vi "Powerstage_Relay_test_v1.vi"() -> ()   [LabVIEW 2022 SP3]
uses:
  <vilib>/DAQmx/read.llb/DAQmx Read (Digital 1D Bool NChan 1Samp 1Line).vi
  <vilib>/DAQmx/miscellaneous.llb/DAQmx Fill In Error Info.vi
panel:
  out "error out":errorcluster
  in  "error in (no error)":errorcluster
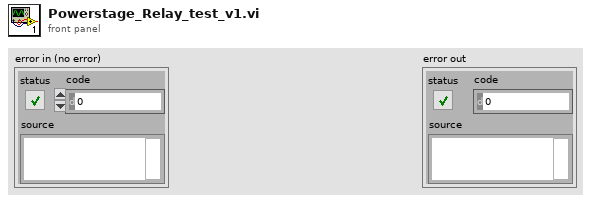
[diagram p1: front panel]
types:
  T1 = cluster{"Set":string, "State on":string, "State off":string}[]
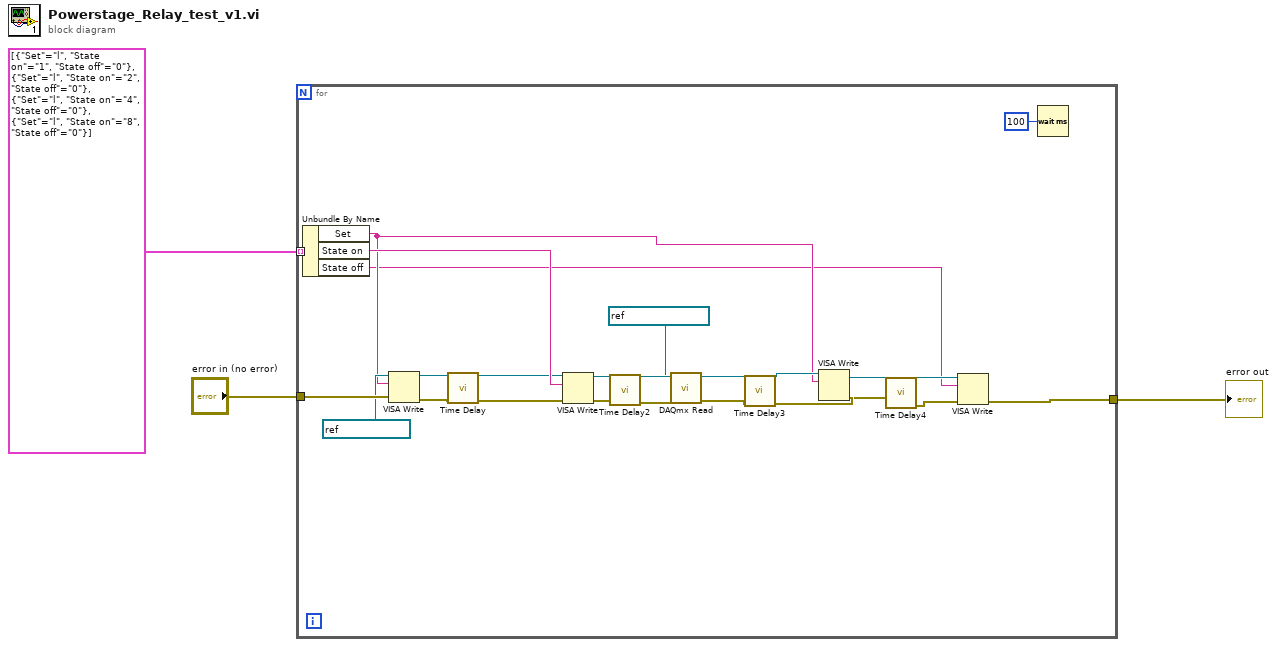
[diagram p0: block diagram]
diagram:
  n1 = for {
    tunnel: T1 [{"Set"="l", "State on"="1", "State off"="0"}, {"Set"="l", "State on"="2", "State off"="0"}, {"Set"="l", "State on"="4", "State off"="0"}, {"Set"="l", "State on"="8", "State off"="0"}] -> [w23] mode=indexing
    tunnel: "error in (no error)" -> [w21]
    tunnel: [w7] -> w1
    n2 = Unbundle By Name(w23) -> ("Set"=w5:string, "State on"=w20:string, "State off"=w4:string)
    n3 = VISA Write(VISA resource name=refnum<visa-resource-name> "ControlBoard", write buffer=w5, error in (no error)=w21) -> (VISA resource name out=w17:refnum<visa-resource-name>, error out=w19:errorcluster)  [unwired: 1 out]
    n4 = call "Time Delay"("error in (no error)"=w19) -> ("error out"=w16:errorcluster)  [unwired: 10 in]
    n5 = VISA Write(VISA resource name=w17, write buffer=w20, error in (no error)=w16) -> (VISA resource name out=w13:refnum<visa-resource-name>, error out=w15:errorcluster)  [unwired: 1 out]
    n6 = call "Time Delay2"("error in (no error)"=w15) -> ("error out"=w14:errorcluster)  [unwired: 10 in]
    n7 = call-poly <vilib>:"DAQmx Read.vi"("task/channels in"=refnum<k21> "FTS2_DigitalIn", "error in"=w14) -> ("error out"=w12:errorcluster)  [unwired: 11 in, 2 out]
    n8 = call "Time Delay3"("error in (no error)"=w12) -> ("error out"=w11:errorcluster)  [unwired: 10 in]
    n9 = VISA Write(VISA resource name=w13, write buffer=w5, error in (no error)=w11) -> (VISA resource name out=w6:refnum<visa-resource-name>, error out=w9:errorcluster)  [unwired: 1 out]
    n10 = call "Time Delay4"("error in (no error)"=w9) -> ("error out"=w8:errorcluster)  [unwired: 10 in]
    n11 = VISA Write(VISA resource name=w6, write buffer=w4, error in (no error)=w8) -> (error out=w7:errorcluster)  [unwired: 2 out]
    n12 = Wait (ms)(milliseconds to wait=u32 100) -> ()  [unwired: 1 out]
  }
  "error out" <- w1
